vi "CreateEvents.vi"(8 "error in (no error)":errorcluster, 11 "NewTemplate in":refnum<class "Layout.lvclass">) -> (0 "error out":errorcluster, 3 "NewTemplate out":refnum<class "Layout.lvclass">)   [LabVIEW 2024, in "Layout.lvclass"]
uses:
  Layout.lvclass
  Layout.lvclass/Layout.ctl
  RQMHCore/ModuleCore/Module.lvclass
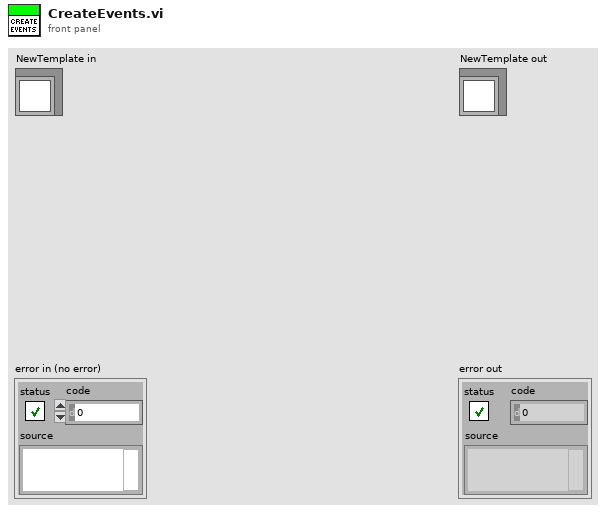
[diagram p1: front panel]
types:
  T1 = typedef "Layout.lvclass/Broadcast Events--cluster.ctl" = cluster{"Stopped":refnum<user-event>}
  T2 = typedef "Layout.lvclass/Request Events--cluster.ctl" = cluster{"Do Something":refnum<user-event>, "Get SubPanel":refnum<user-event>}
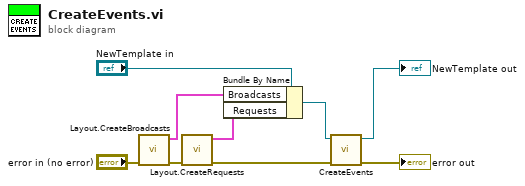
[diagram p0: block diagram]
diagram:
  n1 = call "Layout.CreateBroadcasts.vi"("error in (no error)"="error in (no error)") -> ("error out"=w3:errorcluster, "Broadcasts"=w1:T1)  [unwired: 9 in]
  n2 = call "Layout.CreateRequests.vi"("error in (no error)"=w3) -> ("error out"=w2:errorcluster, "Requests"=w4:T2)  [unwired: 9 in]
  n3 = Bundle By Name(cluster="NewTemplate in", "Broadcasts"=w1, "Requests"=w4) -> (w6:refnum<class "Layout.lvclass">)
  n4 = call-parent "CreateEvents.vi"("error in (no error)"=w2, "JQMHCore in"=w6) -> ("error out"=→"error out":errorcluster, "JQMHCore out"=→"NewTemplate out":refnum<class "Layout.lvclass">)  [unwired: 8 in]
